vi "Classes Destruction.vi"(7 "class labels":T2, 8 "error in":errorcluster, 11 "objects":T1) -> (0 "error out":errorcluster, 3 "objects":T1)   [LabVIEW 2011]
uses:
  Controls/Class Labels.ctl
  Controls/Class Objects.ctl
  Modules/File/Configuration/Configuration.lvclass
  Modules/Hardware/Power Supply/Power Supply.lvclass
  Modules/Hardware/NMR/NMR.lvclass
  Modules/File/TDMS/TDMS.lvclass
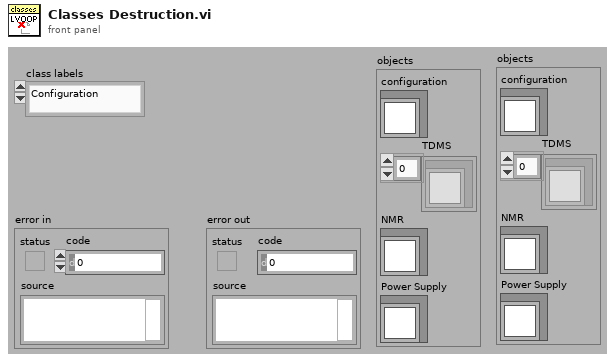
[diagram p1: front panel]
types:
  T1 = typedef "Class Objects.ctl" = cluster{"configuration":refnum<class "Configuration.lvclass">, "TDMS":refnum<class "TDMS.lvclass">[], "Power Supply":refnum<class "Power Supply.lvclass">, "NMR":refnum<class "NMR.lvclass">}
  T2 = typedef "Class Labels.ctl" = enum16{"Configuration", "TDMS", "Detector", "Power Supply", "MFC", "NMR", "Valve Controller"}
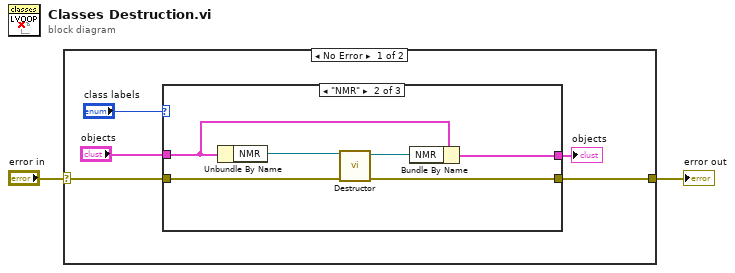
[diagram p0: block diagram]
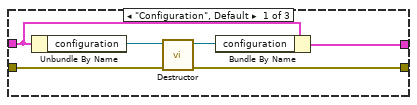
[diagram p2: hidden frame]
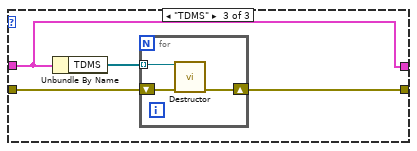
[diagram p3: hidden frame]
diagram:
  n1 = case shown="No Error" "error in" {
    selector: "error in" -> [w6 w27]
    tunnel: [w5 w27] -> w1
    frame No Error {
      n2 = case shown="\"NMR\"" "class labels" {
        tunnel: "objects" -> [w13 w16 w20]
        tunnel: w6 -> [w10 w19 w23]
        tunnel: [w9 w18 w21] -> w5
        tunnel: [w8 w14 w20] -> w3
        frame "Configuration", Default {
          n3 = Unbundle By Name(w13) -> ("configuration"=w12:refnum<class "Configuration.lvclass">)
          n4 = call-dynamic "Destructor.vi"("error in (no error)"=w10, "Configuration in"=w12) -> ("error out"=w9:errorcluster, "Configuration out"=w11:refnum<class "Configuration.lvclass">)  [unwired: 8 in]
          n5 = Bundle By Name(cluster=w13, "configuration"=w11) -> (w8:T1)
        }
        frame "NMR" {
          n6 = Unbundle By Name(w16) -> ("NMR"=w17:refnum<class "NMR.lvclass">)
          n7 = call-dynamic "Destructor.vi"("error in (no error)"=w19, "NMR in"=w17) -> ("error out"=w18:errorcluster, "NMR out"=w15:refnum<class "NMR.lvclass">)  [unwired: 8 in]
          n8 = Bundle By Name(cluster=w16, "NMR"=w15) -> (w14:T1)
        }
        frame "TDMS" {
          n9 = Unbundle By Name(w20) -> ("TDMS"=w22:refnum<class "TDMS.lvclass">[])
          n10 = for {
            shift-right: [w24] -> w21
            shift-left: w23 -> [w26]
            tunnel: w22 -> [w25] mode=indexing
            n11 = call-dynamic "Destructor.vi"("error in"=w26, "TDMS in"=w25) -> ("error out"=w24:errorcluster)  [unwired: 8 in, 1 out]
          }
        }
      }
      "objects" <- w3
    }
    frame Error {
    }
  }
  "error out" <- w1
